vi "DebugCam_Open.vi"(8 "error in (no error)":errorcluster, 9 "h":i32=320, 10 "w":i32=480, 11 "camnum":i32) -> (0 "error out":errorcluster, 3 "status":i32)   [LabVIEW 2014, in "QwaveSys RPi Training Library.lvlib"]
uses:
  <vilib>/Q-Wave Systems/QwaveSys RPi Training Package (Demo)/Addons/QwaveSys RPi Training Library.lvlib
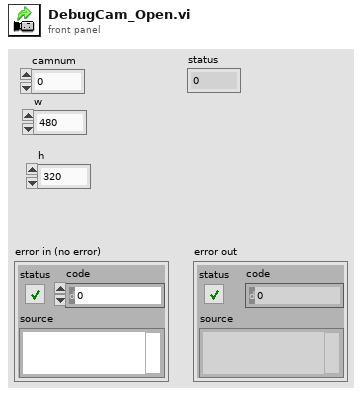
[diagram p1: front panel]
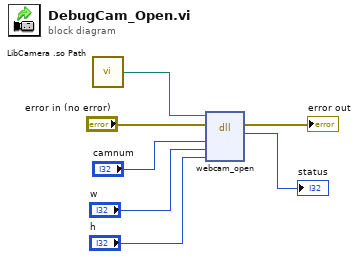
[diagram p0: block diagram]
diagram:
  n1 = call <vilib>:"LibCamera .so Path.vi"() -> ("LibCam .so Path"=w3:path)  [unwired: 5 in]
  n2 = dll-call lib="libcamera.so" fn="webcam_open"(path in=w3, error in="error in (no error)", "camnum"="camnum", "w"="w", "h"="h") -> (error out=→"error out":errorcluster, "return type"=→"status":i32)  [unwired: 4 in, 1 out]
